vi "ParseArgumentsCore.vi"(8 "error in (no error)":errorcluster, 10 "Inputs":string[](array[string]), 11 "MassCompile in":refnum<class "MassCompile.lvclass">) -> (0 "error out":errorcluster, 3 "MassCompile out":refnum<class "MassCompile.lvclass">)   [LabVIEW 2014, in "MassCompile.lvclass"]
uses:
  MassCompile.lvclass
  Utilities/OperationErrorType.ctl
  MassCompile.lvclass/MassCompile.ctl
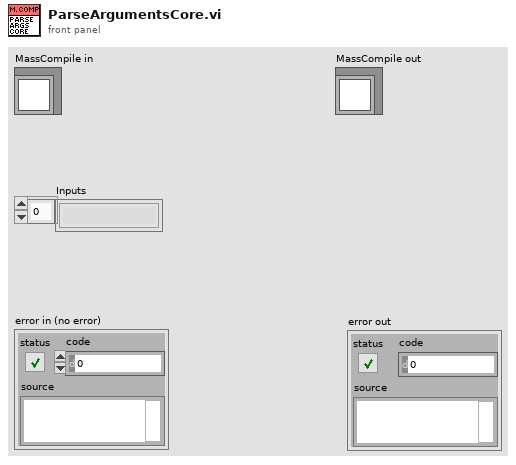
[diagram p1: front panel]
types:
  T1 = typedef "OperationErrorType.ctl" = enum16{"RequiredArgumentMissing", "UnknownArguments", "LoggerSetMultipleTimes", "OperationBrokenError"}
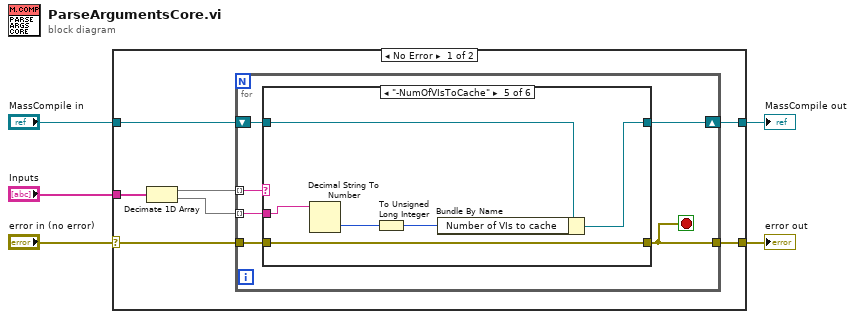
[diagram p0: block diagram]
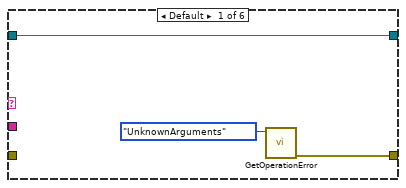
[diagram p2: hidden frame]
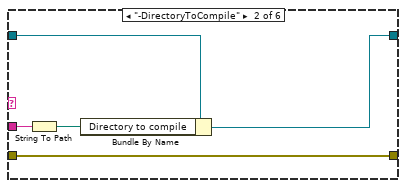
[diagram p3: hidden frame]
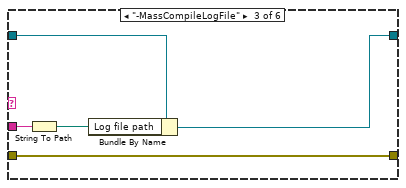
[diagram p4: hidden frame]
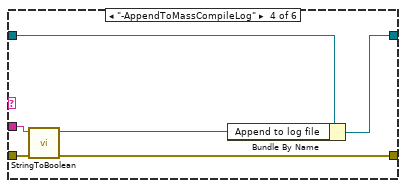
[diagram p5: hidden frame]
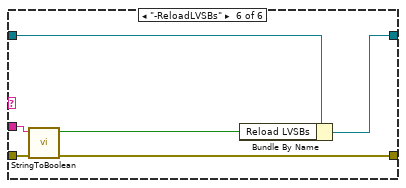
[diagram p6: hidden frame]
diagram:
  n1 = case shown="No Error" "error in (no error)" {
    selector: "error in (no error)" -> [w7 w50]
    tunnel: "MassCompile in" -> [w8 w51]
    tunnel: "Inputs" -> [w12 _]
    tunnel: [w9 w51] -> w4
    tunnel: [w6 w50] -> w5
    frame No Error {
      n2 = Decimate 1D Array(w12) -> (w11:string[], w10:string[])
      n3 = for {
        tunnel: w11 -> [w18] mode=indexing
        tunnel: w10 -> [w17] mode=indexing
        shift-right: [w16] -> w9
        shift-left: w8 -> [w15]
        tunnel: w7 -> [w14]
        tunnel: [w13] -> w6
        stop <- w13 stop-if-true
        n4 = case shown="\"-NumOfVIsToCache\"" w18 {
          tunnel: w17 -> [_ w24 w29 w32 w41 w46]
          tunnel: [w21 w26 w27 w37 w42 w48] -> w16
          tunnel: w15 -> [w21 w25 w31 w33 w43 w49]
          tunnel: [w20 w22 w28 w34 w40 w45] -> w13
          tunnel: w14 -> [_ w22 w28 w35 w40 w44]
          frame Default {
            n5 = call "GetOperationError.vi"("Operation Error Type"=OperationErrorType."UnknownArguments") -> ("error out"=w20:errorcluster)  [unwired: 10 in]
          }
          frame "-DirectoryToCompile" {
            n6 = String To Path(string=w24) -> (path=w23:path)
            n7 = Bundle By Name(cluster=w25, "Directory to compile"=w23) -> (w26:refnum<class "MassCompile.lvclass">)
          }
          frame "-MassCompileLogFile" {
            n8 = String To Path(string=w29) -> (path=w30:path)
            n9 = Bundle By Name(cluster=w31, "Log file path"=w30) -> (w27:refnum<class "MassCompile.lvclass">)
          }
          frame "-AppendToMassCompileLog" {
            n10 = call "StringToBoolean.vi"("error in (no error)"=w35, "Input"=w32) -> ("error out"=w34:errorcluster, "Boolean"=w36:bool)  [unwired: 8 in]
            n11 = Bundle By Name(cluster=w33, "Append to log file"=w36) -> (w37:refnum<class "MassCompile.lvclass">)
          }
          frame "-NumOfVIsToCache" {
            n12 = Decimal String To Number(string=w41) -> (number=w39:i32)  [unwired: 2 in, 1 out]
            n13 = To Unsigned Long Integer(number=w39) -> (unsigned 32bit integer=w38:u32)
            n14 = Bundle By Name(cluster=w43, "Number of VIs to cache"=w38) -> (w42:refnum<class "MassCompile.lvclass">)
          }
          frame "-ReloadLVSBs" {
            n15 = call "StringToBoolean.vi"("error in (no error)"=w44, "Input"=w46) -> ("error out"=w45:errorcluster, "Boolean"=w47:bool)  [unwired: 8 in]
            n16 = Bundle By Name(cluster=w49, "Reload LVSBs"=w47) -> (w48:refnum<class "MassCompile.lvclass">)
          }
        }
      }
    }
    frame Error {
    }
  }
  "error out" <- w5
  "MassCompile out" <- w4
